vi "pf_Camera_Properties_manager.vi"(7 "Action":T4=enum."Get", 8 "error in (no error)":errorcluster, 9 "Properties Array":T1[](array[typedef]), 11 "IMAQ Session in":refnum<k11>) -> (0 "error out":errorcluster, 1 "Properties Array out":T1[](array[typedef]), 3 "IMAQ Session out":refnum<k11>)   [LabVIEW 2025, in "Photonfocus_Toolkit.lvlib"]
doc: "manages all the parameters needed by the library."
uses:
  Photonfocus_Toolkit.lvlib
  Controls/pf_Camera_ctrl_mngr_action.ctl
  Controls/pf_Property_Cluster.ctl
  Controls/pf_Property_Type.ctl
  Controls/pf_Property_Flag.ctl
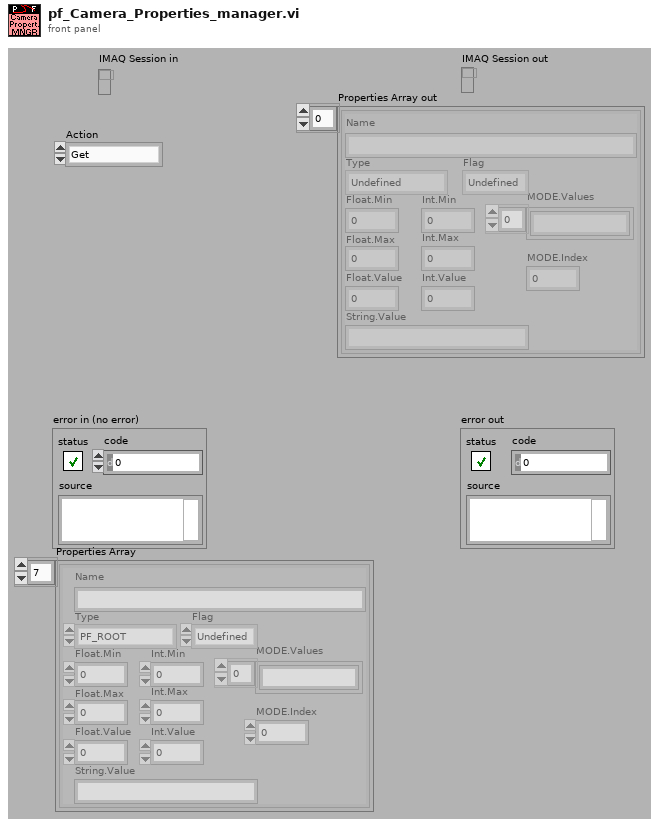
[diagram p1: front panel]
types:
  T1 = typedef "Photonfocus_Toolkit.lvlib/pf_Property_Cluster.ctl" = cluster{"Name":string, "Type":T2, "Float.Min":sgl, "Float.Max":sgl, "Float.Value":sgl, "Int.Min":u32, "Int.Max":u32, "Int.Value":u32, "String.Value":string, "MODE.Values":string[], "MODE.Index":i32, "Flag":T3}
  T2 = typedef "Photonfocus_Toolkit.lvlib/pf_Property_Type.ctl" = enum16{"Undefined", "PF_ROOT", "PF_INT", "PF_FLOAT", "PF_BOOL", "PF_MODE", "PF_REGISTER", "PF_STRING", "PF_BUFFER", "PF_STRUCT", "PF_ARRAY", "PF_COMMAND", "PF_EVENT"}
  T3 = typedef "Photonfocus_Toolkit.lvlib/pf_Property_Flag.ctl" = enum16{"Undefined", "RO", "WO", "RW"}
  T4 = typedef "Photonfocus_Toolkit.lvlib/pf_Camera_ctrl_mngr_action.ctl" = enum16{"Create", "Destroy", "Set", "Get"}
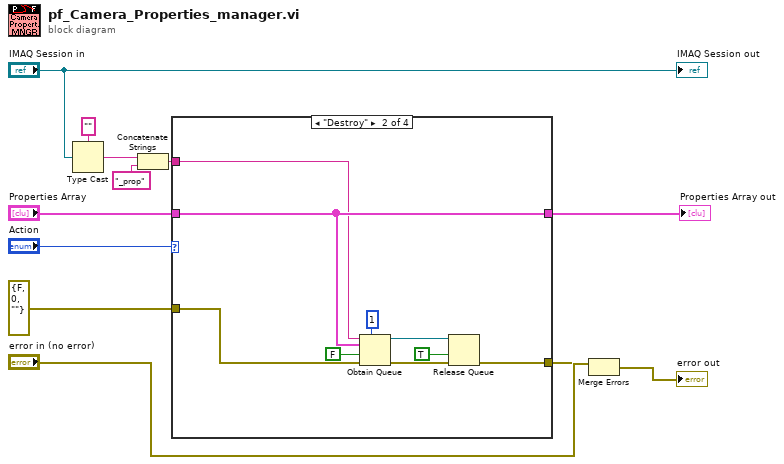
[diagram p0: block diagram]
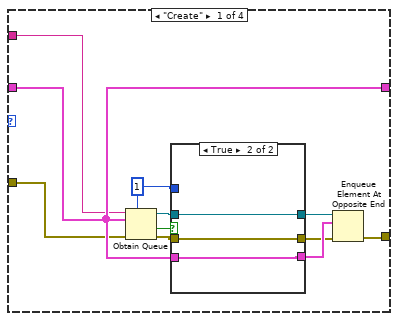
[diagram p2: hidden frame]
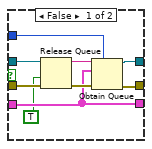
[diagram p3: hidden frame]
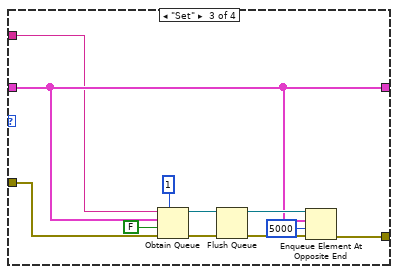
[diagram p4: hidden frame]
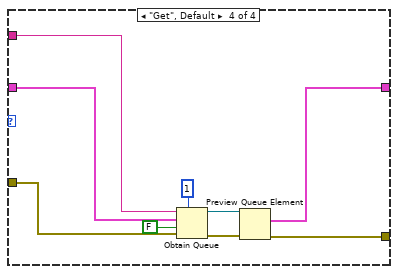
[diagram p5: hidden frame]
diagram:
  n1 = Type Cast(type="", x="IMAQ Session in") -> (*(type *) &x=w2:string)
  n2 = Concatenate Strings(w2, "_prop" ("string")) -> (w5:string)
  n3 = case shown="\"Destroy\"" "Action" {
    tunnel: [w19 w37 w55 w59] -> w9
    tunnel: [w15 w40 w48 w60] -> w6
    tunnel: "Properties Array" -> [w15 w40 w48 w58]
    tunnel: errorcluster {"status"=FALSE, "code"=0, "source"=""} ("error in (no error)") -> [w14 w38 w46 w57]
    tunnel: w5 -> [w13 w36 w45 w56]
    frame "Create" {
      w18 = 1 ("max queue size (-1, unlimited)")
      n4 = Obtain Queue(max queue size (-1, unlimited)=w18, name (unnamed)=w13, element data type=w15, error in (no error)=w14) -> (queue out=w17:refnum<queue>, created new?=w16:bool, error out=w20:errorcluster)  [unwired: 1 in]
      n5 = case shown="True" w16 {
        tunnel: w20 -> [w32 w35]
        tunnel: [w27 w35] -> w21
        tunnel: w17 -> [w31 w34]
        tunnel: w18 -> [w28 _]
        tunnel: w15 -> [w25 w33]
        tunnel: [w26 w34] -> w22
        tunnel: [w25 w33] -> w23
        frame False {
          n6 = Release Queue(queue=w31, force destroy? (F)=TRUE, error in (no error)=w32) -> (queue name=w29:string, error out=w30:errorcluster)  [unwired: 1 out]
          n7 = Obtain Queue(max queue size (-1, unlimited)=w28, name (unnamed)=w29, element data type=w25, error in (no error)=w30) -> (queue out=w26:refnum<queue>, error out=w27:errorcluster)  [unwired: 1 in, 1 out]
        }
        frame True {
        }
      }
      n8 = Enqueue Element At Opposite End(queue=w22, element=w23, error in (no error)=w21) -> (error out=w19:errorcluster)  [unwired: 3 out]
    }
    frame "Destroy" {
      n9 = Obtain Queue(max queue size (-1, unlimited)=1, name (unnamed)=w36, element data type=w40, create if not found? (T)=FALSE, error in (no error)=w38) -> (queue out=w41:refnum<queue>, error out=w44:errorcluster)  [unwired: 1 out]
      n10 = Release Queue(queue=w41, force destroy? (F)=TRUE, error in (no error)=w44) -> (error out=w37:errorcluster)  [unwired: 2 out]
    }
    frame "Set" {
      n11 = Obtain Queue(max queue size (-1, unlimited)=1, name (unnamed)=w45, element data type=w48, create if not found? (T)=FALSE, error in (no error)=w46) -> (queue out=w51:refnum<queue>, error out=w52:errorcluster)  [unwired: 1 out]
      n12 = Flush Queue(queue=w51, error in (no error)=w52) -> (queue out=w50:refnum<queue>, error out=w49:errorcluster)  [unwired: 1 out]
      n13 = Enqueue Element At Opposite End(queue=w50, element=w48, timeout in ms (-1)=5000, error in (no error)=w49) -> (error out=w55:errorcluster)  [unwired: 2 out]
    }
    frame "Get", Default {
      n14 = Obtain Queue(max queue size (-1, unlimited)=1, name (unnamed)=w56, element data type=w58, create if not found? (T)=FALSE, error in (no error)=w57) -> (queue out=w62:refnum<queue>, error out=w64:errorcluster)  [unwired: 1 out]
      n15 = Preview Queue Element(queue=w62, error in (no error)=w64) -> (element=w60:T1[], error out=w59:errorcluster)  [unwired: 3 out]
    }
  }
  "Properties Array out" <- w6
  n16 = Merge Errors("error in (no error)", w9) -> (→"error out":errorcluster)
  "IMAQ Session out" <- "IMAQ Session in"
